vi "ButtonPickUpBarrel.vi"(11 "Buttons":bool[](array[boolean])) -> ()   [LabVIEW 2014]
uses:
  FeederStationPickup.ctl
  Gantry/GantryGlobals.vi
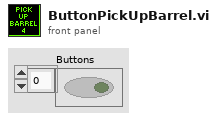
[diagram p1: front panel]
types:
  T1 = typedef "FeederStationPickup.ctl" = enum16{"WaitingForInput", "LiftTo2Totes", "CloseArms", "LiftTo4Totes", "ReleaseArms"}
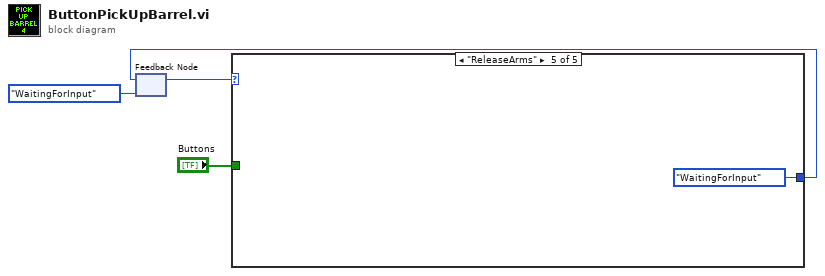
[diagram p0: block diagram]
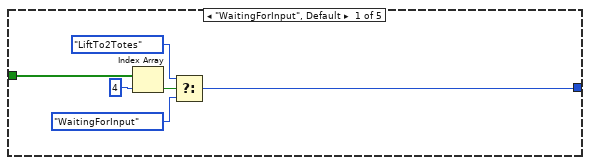
[diagram p2: hidden frame]
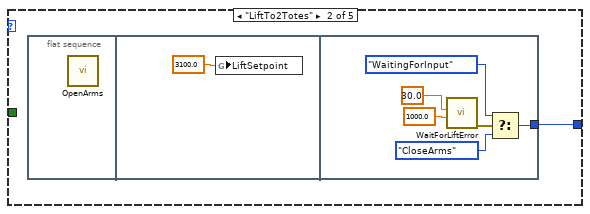
[diagram p3: hidden frame]
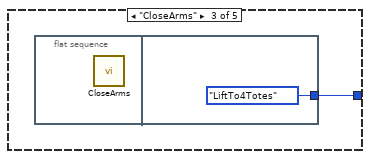
[diagram p4: hidden frame]
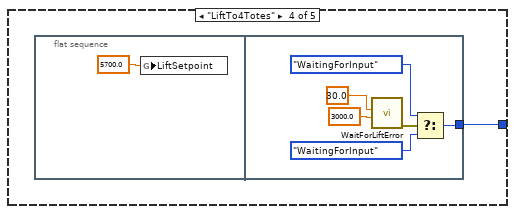
[diagram p5: hidden frame]
diagram:
  n1 = feedback #1(FeederStationPickup."WaitingForInput" ("FeederStationPickup")) -> (w2:T1)
  n2 = case shown="\"ReleaseArms\"" w2 {
    tunnel: [w7 w11 w19 w21 FeederStationPickup."WaitingForInput" ("FeederStationPickup")] -> w3
    tunnel: "Buttons" -> [w6 _ _ _ _]
    frame "WaitingForInput", Default {
      n3 = Index Array(array=w6, index=4) -> (element=w5:bool)
      n4 = Select(t=FeederStationPickup."LiftTo2Totes" ("FeederStationPickup"), s=w5, f=FeederStationPickup."WaitingForInput" ("FeederStationPickup")) -> (s? t:f=w7:T1)
    }
    frame "LiftTo2Totes" {
      n5 = flat-sequence {
        tunnel: [w13] -> w11
        frame #0 {
          n6 = call "OpenArms.vi"() -> ()  [unwired: 12 in]
        }
        frame #1 {
          n7 = global write "GantryGlobals.vi" "LiftSetpoint"(3100.0 ("LiftSetpoint")) -> ()
        }
        frame #2 {
          n8 = call "WaitForLiftError.vi"("Timeout (ms)"=1000.0, "AllowedError"=30.0) -> ("error out"=w16:errorcluster)  [unwired: 9 in]
          n9 = Select(t=FeederStationPickup."WaitingForInput" ("FeederStationPickup"), s=w16, f=FeederStationPickup."CloseArms" ("FeederStationPickup")) -> (s? t:f=w13:T1)
        }
      }
    }
    frame "CloseArms" {
      n10 = flat-sequence {
        tunnel: [FeederStationPickup."LiftTo4Totes" ("FeederStationPickup")] -> w19
        frame #0 {
          n11 = call "CloseArms.vi"() -> ()  [unwired: 12 in]
        }
        frame #1 {
        }
      }
    }
    frame "LiftTo4Totes" {
      n12 = flat-sequence {
        tunnel: [w23] -> w21
        frame #0 {
          n13 = global write "GantryGlobals.vi" "LiftSetpoint"(5700.0 ("LiftSetpoint")) -> ()
        }
        frame #1 {
          n14 = call "WaitForLiftError.vi"("Timeout (ms)"=3000.0, "AllowedError"=30.0) -> ("error out"=w28:errorcluster)  [unwired: 9 in]
          n15 = Select(t=FeederStationPickup."WaitingForInput" ("FeederStationPickup"), s=w28, f=FeederStationPickup."WaitingForInput" ("FeederStationPickup")) -> (s? t:f=w23:T1)
        }
      }
    }
    frame "ReleaseArms" {
    }
  }
  n16 = feedback-in #1(w3) -> ()
